vi "gl_Initialise_Images.vi"() -> (3 "Live image refs":T1)   [LabVIEW 2013]
uses:
  User Interface/Queue/Live graphs queue/Typedefs/Live imaging queue element.ctl
  <vilib>/vision/Image Controls.llb/IMAQ Image.ctl
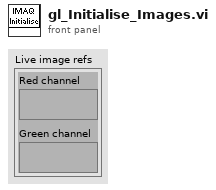
[diagram p1: front panel]
types:
  T1 = typedef "Live imaging queue element.ctl" = cluster{"Red channel":T2, "Green channel":T2}
  T2 = typedef "IMAQ Image.ctl" = refnum<image>
  T3 = typedef "Image Type" = u32
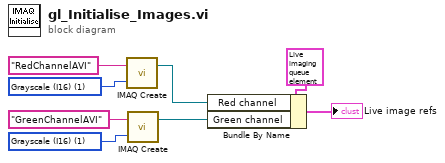
[diagram p0: block diagram]
diagram:
  w8 = T3 1 items=["Grayscale (U8)", "Grayscale (I16)", "Grayscale (SGL)", "Complex (CSG)", "RGB (U32)", "HSL (U32)", "RGB (U64)", "Grayscale (U16)"] ("Image Type")
  w5 = T3 1 items=["Grayscale (U8)", "Grayscale (I16)", "Grayscale (SGL)", "Complex (CSG)", "RGB (U32)", "HSL (U32)", "RGB (U64)", "Grayscale (U16)"] ("Image Type")
  n1 = call "IMAQ Create"("Image Name"="RedChannelAVI", "Image Type"=w8) -> ("New Image"=w3:T2)  [unwired: 3 in, 1 out]
  n2 = call "IMAQ Create"("Image Name"="GreenChannelAVI", "Image Type"=w5) -> ("New Image"=w2:T2)  [unwired: 3 in, 1 out]
  n3 = Bundle By Name(cluster=T1 {"Red channel"=refnum, "Green channel"=refnum} ("Element to queue"), "Red channel"=w3, "Green channel"=w2) -> (→"Live image refs":T1)
